vi "Read With Abort.vi"(6 "abort":bool, 7 "timeout in ms (0)":i32, 10 "channel":T1) -> (2 "element":T2={"Temp. Sensirion"=0.01, "Hum. Sensirion"=0.01, "Temp. Switch Matrix"=0.01, "Hum. Switch Matrix"=0.01, "Temp. Probecard"=0.01, "Hum. Probecard"=0.01} {"Hum. Probecard" format="%#_13g"; "Temp. Probecard" format="%#_13g"; "Hum. Switch Matrix" format="%#_13g"; "Temp. Switch Matrix" format="%#_13g"; "Hum. Sensirion" format="%#_13g"; "Temp. Sensirion" format="%#_13g"}, 4 "aborted?":bool, 5 "missed":i32)   [LabVIEW 2020, in "Tag-t'data_env.ctl'.lvlib"]
doc: "Reads a value from a Tag channel or signals the channel to abort. This endpoint is the same as the Read endpoint except that it has an <B>abort</B> input and an <B>aborted?</B> output. You can use the abort capability of the Tag channel to close a channel abruptly, ignoring any data left in the channel buffer. You must use this endpoint together with the Write With Abort endpoint."
uses:
  <extravilib>/ChannelInstances/Tag-t'data_env.ctl'.lvlib
  Desktop/HexDAQ/src/data_env.ctl
  <extravilib>/ChannelInstances/Tag-t'data_env.ctl'/))Channel.ctl
panel:
  # "number of values missed\n(-1 means element is stale or timed out)"
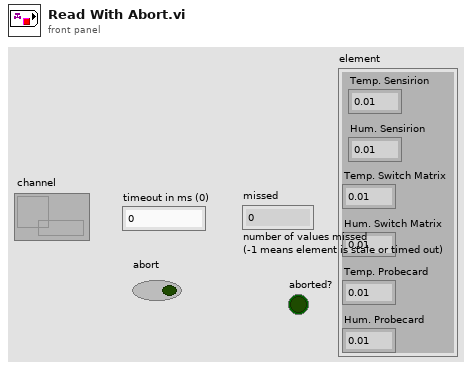
[diagram p1: front panel]
types:
  T1 = typedef "Tag-t'data_env.ctl'.lvlib/))Channel.ctl" = refnum<queue>
  T2 = typedef "data_env.ctl" = cluster{"Temp. Sensirion":dbl, "Hum. Sensirion":dbl, "Temp. Switch Matrix":dbl, "Hum. Switch Matrix":dbl, "Temp. Probecard":dbl, "Hum. Probecard":dbl}
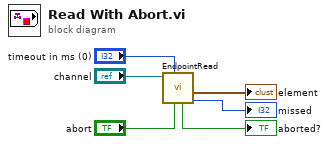
[diagram p0: block diagram]
diagram:
  n1 = call <extravilib>:"EndpointRead.vi"("abort (F)"="abort", "timeout in ms (-1)"="timeout in ms (0)", "channel in"="channel") -> ("missed"=→"missed":i32, "element out"=→"element":T2, "aborted?"=→"aborted?":bool)  [unwired: 5 in, 1 out]
